vi "3-Fibonacci Numbers.vi"() -> ()   [LabVIEW 2015]
panel:
  out "XY Graph":cluster{i32[], i32[]}(graph)
  in  "Stop":bool
  out "Fibonacci Function-F(x)":u32
  in  "n. Term":i32
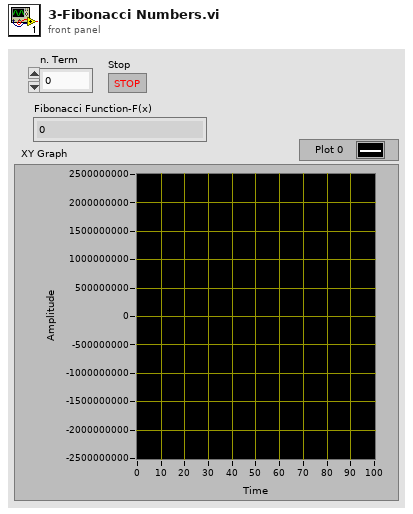
[diagram p1: front panel]
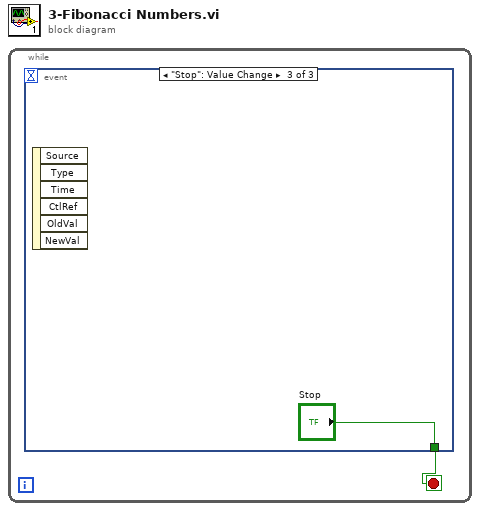
[diagram p0: block diagram]
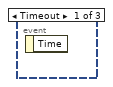
[diagram p2: hidden frame]
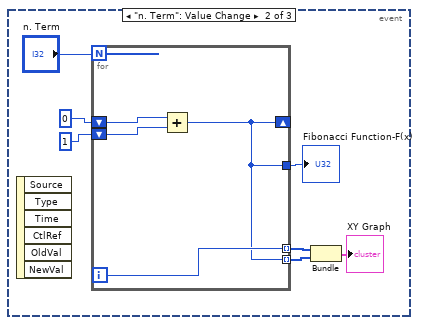
[diagram p3: hidden frame]
diagram:
  n1 = while {
    stop <- w1 stop-if-true
    n2 = event shown="[2] \"Stop\": Value Change" {
      selector: _ -> [_ _ _]
      dyn-events: _ -> [_ _ _]
      timeout: _ -> [_ _ _]
      tunnel: [_ _ "Stop"] -> w1
      event Timeout {
        n3 = event-data() -> ()  [unwired: 1 in, 1 out]
      }
      event "n. Term": Value Change {
        n4 = event-data() -> ()  [unwired: 1 in, 6 out]
        n5 = for {
          N: "n. Term" -> [_]
          shift-right: [w9] -> _
          shift-left: 0 -> [w12]
          shift-left: 1 -> [w10]
          tunnel: [w11] -> w7 mode=indexing
          tunnel: [w9] -> w5 mode=indexing
          tunnel: [w9] -> w4
          i -> [w11]
          n6 = Add(x=w12, y=w10) -> (x+y=w9:i32)
        }
        "Fibonacci Function-F(x)" <- w4
        n7 = Bundle(w7, w5) -> (→"XY Graph":cluster{i32[], i32[]})  [unwired: 1 in]
      }
      event "Stop": Value Change {
        n8 = event-data() -> ()  [unwired: 1 in, 6 out]
      }
    }
  }
